vi "releaseQueue.vi"(8 "error in (no error)":errorcluster, 11 "TCPCommunicator in":refnum<class "TCPCommunicator.lvclass">) -> (0 "error out":errorcluster, 3 "TCPCommunicator out":refnum<class "TCPCommunicator.lvclass">)   [LabVIEW 2016, in "TCPCommunicator.lvclass"]
uses:
  TCPCommunicator.lvclass
  TCPCommunicator.lvclass/TCPCommunicator.ctl
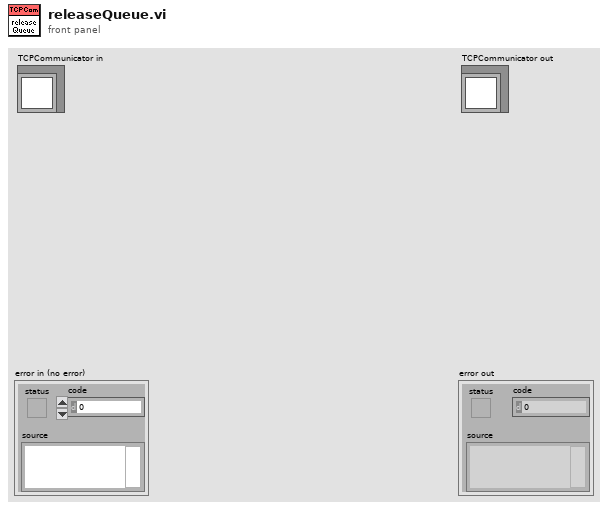
[diagram p1: front panel]
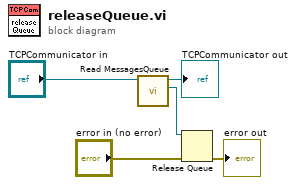
[diagram p0: block diagram]
diagram:
  n1 = call "Read MessagesQueue.vi"("TCPCommunicator in"="TCPCommunicator in") -> ("MessagesQueue"=w5:refnum<queue>, "TCPCommunicator out"=→"TCPCommunicator out":refnum<class "TCPCommunicator.lvclass">)  [unwired: 8 in, 1 out]
  n2 = Release Queue(queue=w5, error in (no error)="error in (no error)") -> (error out=→"error out":errorcluster)  [unwired: 1 in, 2 out]
